vi "test-SetGetControlValues.vi"() -> (0 "Result":errorcluster[](array[cluster]))   [LabVIEW 2019]
panel:
  in  "Array of Cluster":cluster{"Weired//=|\"Name\" //[2]":dbl}[](array[cluster])
  in  "String":string
  in  "Numeric":dbl
  in  "Array":T1(array[cluster])=[{"Set"="test-SetGetControlValues\nNumeric=1\nString=\"aa\"\nArray of Cluster=[{0:1},{0:2},{0:3}]\n\ntest-controls\nDouble=1.1", "Get"="test-SetGetControlValues\nNumeric\nString\n// コメントを入れられる\nArray of Cluster\n\ntest-controls\nDouble\n// コメントを入れられる\n", "Expect"="{\"test-SetGetControlValues\":{\"Numeric\":1,\"String\":\"aa\",\"Array of Cluster\":[{\"Weired//=|\\\"Name\\\" //[2]\":1},{\"Weired//=|\\\"Name\\\" //[2]\":2},{\"Weired//=|\\\"Name\\\" //[2]\":3}]},\"test-controls\":{\"Double\":1.1}}", "Error"=FALSE, "Result"=""}, {"Set"="test-SetGetControlValues\nArray of Cluster[0]={0:-1}\n\n\n\n//2行以上空いても大丈夫\n//最後に改行がなくても大丈夫\ntest-controls\n// コントロール名が / を含むなら \\/ にエスケープ\nWeired\\/Control\\/Name=3\n// = を含むときも \\= にエスケープ\nWeired\\/Control\\/Name\\=2=-1", "Get"="// 表示名を付けてみる\ntest-SetGetControlValues|this\nArray of Cluster[0]\n\ntest-controls|that\nWeired\\/Control\\/Name|Weired\"\"\n// 読み取りでは = をエスケープしない\nWeired\\/Control\\/Name=2", "Expect"="{\"this\":{\"Array of Cluster[0]\":{\"Weired//=|\\\"Name\\\" //[2]\":-1}},\"that\":{\"Weired\\\"\\\"\":3,\"Weired/Control/Name=2\":-1}}", "Error"=FALSE, "Result"=""}, {"Set"="test-SetGetControlValues\nArray of Cluster[0]/0=0\n// 後ろに余計な空行があっても大丈夫\n\n\n", "Get"="test-SetGetControlValues\nArray of Cluster[0]/0\n", "Expect"="{\"test-SetGetControlValues\":{\"Array of Cluster[0]/0\":0}}", "Error"=FALSE, "Result"=""}, {"Set"="test-SetGetControlValues\nArray of Cluster[0]/Weired\\/\\/\\=\\|\"Name\" \\/\\/\\[2]=5\n// コメントの末尾に改行がなくても大丈夫", "Get"="test-SetGetControlValues\nArray of Cluster[0]/Weired\\/\\/\\=\\|\"Name\" \\/\\/\\[2]|Weired\n// オブジェクトのキーになるときには \\/ のエスケープが失われてしまうのでパスの区切りと区別がつかなくなる", "Expect"="{\"test-SetGetControlValues\":{\"Weired\":5}}", "Error"=FALSE, "Result"=""}, {"Set"="// 元に戻しておく\ntest-SetGetControlValues\nNumeric=0\nString=\"\"\nArray of Cluster=[]", "Get"="// 何も指定しないと空のオブジェクトが返る", "Expect"="{}", "Error"=FALSE, "Result"=""}]
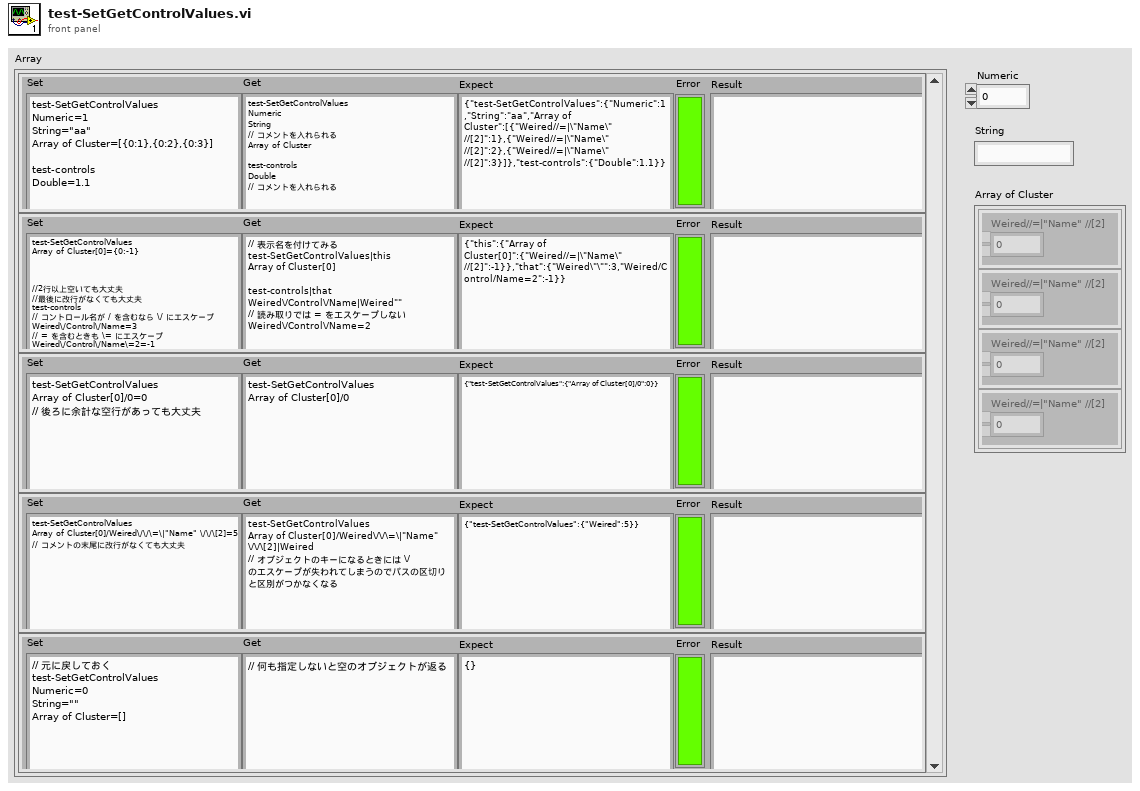
[diagram p1: front panel]
types:
  T1 = cluster{"Set":string, "Get":string, "Expect":string, "Error":bool, "Result":string}[]
  T2 = enum32{"Invalid", "Standard", "Closed", "Hidden", "Minimized", "Maximized"}
  T3 = cluster{"Set":string, "Get":string, "Expect":string, "Error":bool, "Result":string}
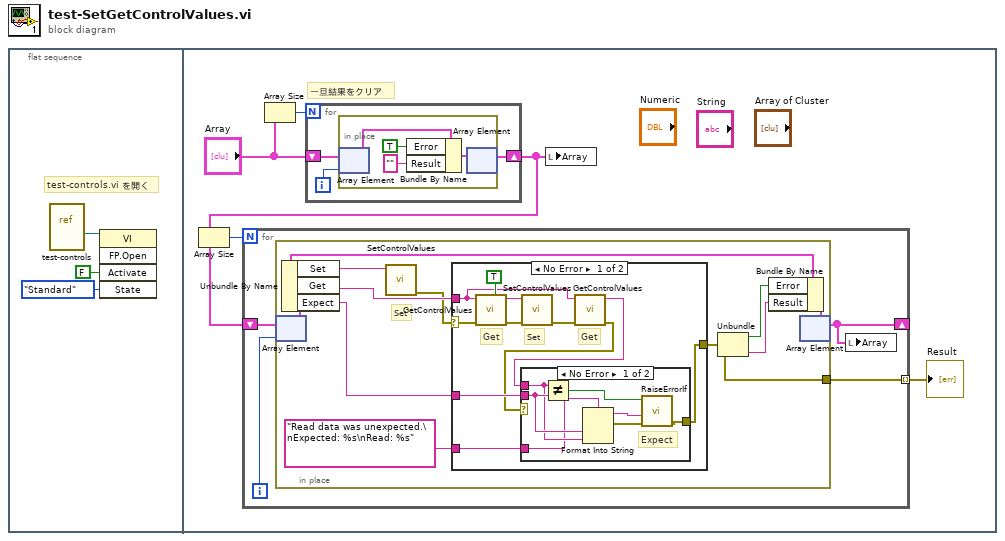
[diagram p0: block diagram]
diagram:
  n1 = flat-sequence {
    frame #0 {
      # "test-controls.vi を開く"
      n2 = vi-ref "test-controls.vi"() -> (w3:refnum<vi>)
      n3 = invoke class="VI" method="FP.Open"(reference=w3, "Activate"=FALSE ("Activate?"), "State"=T2."Standard") -> ()  [unwired: 2 in, 5 out]
    }
    frame #1 {
      # "一旦結果をクリア"
      n4 = Array Size(array="Array") -> (size(s)=w8:i32)
      n5 = for {
        N: w8 -> [_]
        shift-right: [w10] -> w5
        shift-left: "Array" -> [w11]
        i -> [w9]
        n6 = in-place {
          n7 = in-place-array #1(w11, w9) -> (w15:T3)
          n8 = Bundle By Name(cluster=w15, "Error"=TRUE, "Result"="") -> (w14:T3)
          n9 = in-place-array #1(w14) -> (w10:T1)  [unwired: 1 out]
        }
      }
      n10 = Array Size(array=w5) -> (size(s)=w6:i32)
      n11 = for {
        N: w6 -> [_]
        shift-right: [w18] -> _
        shift-left: w5 -> [w19]
        tunnel: [w16] -> w4 mode=indexing
        i -> [w17]
        n12 = in-place {
          in-place-border: [w20] -> w16
          # "Set"
          n13 = in-place-array #2(w19, w17) -> (w29:T3)
          n14 = Unbundle By Name(w29) -> ("Set"=w27:string, "Get"=w26:string, "Expect"=w24:string)
          n15 = call "SetControlValues.vi"("ControlValueList"=w27) -> ("error out"=w25:errorcluster)  [unwired: 10 in]
          n16 = case shown="No Error" w25 {
            selector: w25 -> [w40 w49]
            tunnel: w26 -> [w32 _]
            tunnel: w24 -> [w39 _]
            tunnel: "Read data was unexpected.\nExpected: %s\nRead: %s" -> [w38 _]
            tunnel: [w37 w49] -> w20
            frame No Error {
              # "Get"
              # "Set"
              # "Get"
              n17 = call "GetControlValues.vi"("As List"=TRUE, "error in"=w40, "ControlList"=w32) -> ("error out"=w34:errorcluster, "Control Values"=w35:string)  [unwired: 7 in]
              n18 = call "SetControlValues.vi"("error in"=w34, "ControlValueList"=w35) -> ("error out"=w33:errorcluster)  [unwired: 9 in]
              n19 = call "GetControlValues.vi"("error in"=w33, "ControlList"=w32) -> ("error out"=w30:errorcluster, "Control Values"=w31:string)  [unwired: 8 in]
              n20 = case shown="No Error" w30 {
                selector: w30 -> [_ w48]
                tunnel: w31 -> [w46 _]
                tunnel: w39 -> [w47 _]
                tunnel: w38 -> [w45 _]
                tunnel: [w41 w48] -> w37
                frame No Error {
                  # "Expect"
                  n21 = Not Equal?(x=w46, y=w47) -> (x != y?=w42:bool)
                  n22 = Format Into String(format string=w45, w47, w46) -> (resulting string=w43:string, error out=w44:errorcluster)  [unwired: 2 in]
                  n23 = call "RaiseErrorIf.vi"("error in (no error)"=w44, "error message"=w43, "error? (true)"=w42) -> ("error out"=w41:errorcluster)  [unwired: 8 in]
                }
                frame Error {
                }
              }
            }
            frame Error {
            }
          }
          n24 = Unbundle(w20) -> ("status"=w22:bool, "source"=w21:string)  [unwired: 1 out]
          n25 = Bundle By Name(cluster=w29, "Error"=w22, "Result"=w21) -> (w28:T3)
          n26 = in-place-array #2(w28) -> (w18:T1)  [unwired: 1 out]
        }
        n27 = local write "Array"(w18) -> ()
      }
      "Result" <- w4
      n28 = local write "Array"(w5) -> ()
    }
  }
